vi "event_common_die.vi"(6 "local_common":refnum<user-event>, 8 "error in (no error)":errorcluster) -> (0 "error out":errorcluster)   [LabVIEW 2015, in "lv-interface-sub-re.lvlib"]
uses:
  lv-interface-sub-re.lvlib
  _controls/event_common.ctl
  _controls/event_common_command.ctl
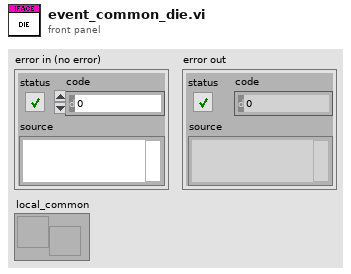
[diagram p1: front panel]
types:
  T1 = typedef "lv-interface-sub-re.lvlib/event_common.ctl" = cluster{"command":T2, "data":variant}
  T2 = typedef "lv-interface-sub-re.lvlib/event_common_command.ctl" = enum16{"<event_common_cmd>", "die", "<null>"}
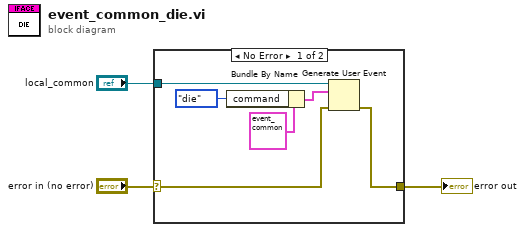
[diagram p0: block diagram]
diagram:
  n1 = case shown="No Error" "error in (no error)" {
    selector: "error in (no error)" -> [w7 w10]
    tunnel: [w9 w10] -> w2
    tunnel: "local_common" -> [w6 _]
    frame No Error {
      n2 = Bundle By Name(cluster=T1 {"command"=enum."<event_common_cmd>", "data"=variant} ("event data"), "command"=event_common_command."die") -> (w4:T1)
      n3 = Generate User Event(user event=w6, event data cluster=w4, error in=w7) -> (error out=w9:errorcluster)  [unwired: 1 in, 1 out]
    }
    frame Error {
    }
  }
  "error out" <- w2
